vi "update_shutter.vi"(5 "commit?":bool, 6 "error in":errorcluster, 7 "Shutter":bool, 8 "TTL external control?":bool, 9 "port in":refnum<visa-resource-name>) -> (0 "error out":errorcluster, 1 "cmd string":string, 2 "disable shutter button?":bool, 3 "port out":refnum<visa-resource-name>, 4 "update COM error status":bool)   [LabVIEW 2016]
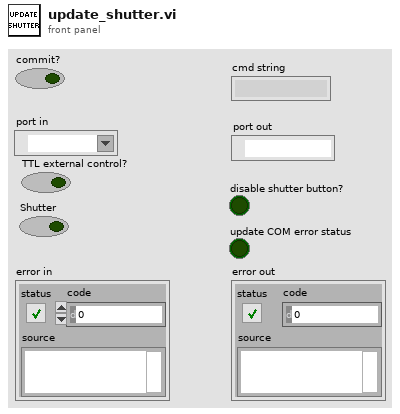
[diagram p1: front panel]
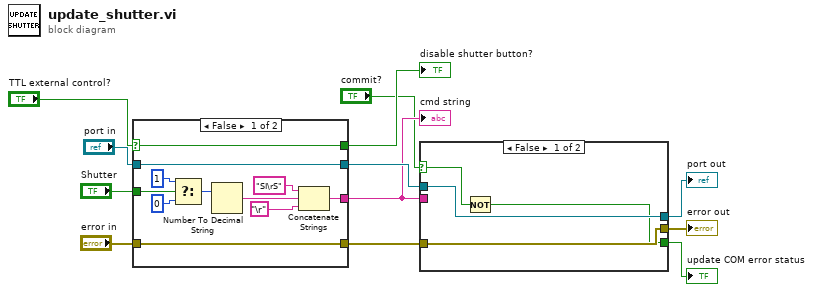
[diagram p0: block diagram]
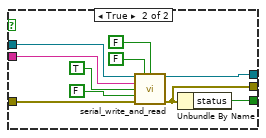
[diagram p2: hidden frame]
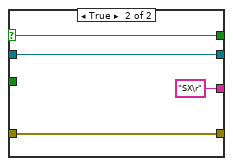
[diagram p3: hidden frame]
diagram:
  n1 = case shown="False" "TTL external control?" {
    selector: "TTL external control?" -> [w20 w27]
    tunnel: "port in" -> [w15 w26]
    tunnel: [w14 w25] -> w5
    tunnel: [w15 w26] -> w4
    tunnel: "error in" -> [w14 w25]
    tunnel: "Shutter" -> [w19 _]
    tunnel: [w20 w27] -> w8
    tunnel: [w13 "SX\r" ("write buffer")] -> w3
    frame False {
      n2 = Select(t=i8 1, s=w19, f=i8 0) -> (s? t:f=w21:i8)
      n3 = Number To Decimal String(number=w21) -> (decimal integer string=w18:string)  [unwired: 1 in]
      n4 = Concatenate Strings("SI\rS" ("string"), w18, "\r") -> (w13:string)
    }
    frame True {
    }
  }
  "disable shutter button?" <- w8
  "cmd string" <- w3
  n5 = case shown="False" "commit?" {
    selector: "commit?" -> [w29 _]
    tunnel: w4 -> [w31 w41]
    tunnel: [w30 w33] -> w7
    tunnel: [w31 w40] -> w6
    tunnel: w5 -> [w30 w39]
    tunnel: w3 -> [_ w38]
    tunnel: [w28 w32] -> w1
    frame False {
      n6 = Not(x=w29) -> (.not. x?=w28:bool)
    }
    frame True {
      n7 = call "serial_write_and_read.vi"("port name in"=w41, "reconnect?"=FALSE, "disconnect?"=FALSE, "write buffer"=w38, "do writing?"=TRUE, "expecting response?"=FALSE, "error in"=w39) -> ("port name out"=w40:refnum<visa-resource-name>, "error out"=w33:errorcluster)  [unwired: 6 in, 1 out]
      n8 = Unbundle By Name(w33) -> ("status"=w32:bool)
    }
  }
  "error out" <- w7
  "port out" <- w6
  "update COM error status" <- w1
